vi "OAT Cascade Plot.vi"(0 "spectral map":dbl[][](array[numeric]) format="%.2f", 1 "cascade plot ref":refnum<vi>, 2 "reset? (F)":bool, 5 "spectral map info":T1={"scales"={"x scale"={"offset"=0.0, "multiplier"=0.0}, "y scale"={"offset"=0.0, "multiplier"=0.0}}, "unit labels"={"x-axis unit label"="", "y-axis unit label"="", "z-axis unit label"=""}, "plot type"=enum."Frequency-Time", "dB on"=TRUE} {"scales"."y scale"."multiplier" format="%.2f"; "scales"."y scale"."offset" format="%.2f"; "scales"."x scale"."multiplier" format="%.2f"; "scales"."x scale"."offset" format="%.2f"}, 9 "order grids to display [order]":dbl[](array[numeric]), 11 "error in (no error)":errorcluster, 12 "plot settings":T2={"plot color"=16860, "grid color"=11776947, "max Z range"=11, "number of spectra"=40} {"max Z range" items=["10^-7", "10^-6", "10^-5", "0.0001", "0.001", "0.01", "0.1", "1", "10", "100", "1000", "auto z range"]}) -> (4 "cascade plot":T3, 15 "error out":errorcluster)   [LabVIEW 2017]
doc: "LabVIEW no longer supports this VI. Use the OAT Spectral Map VI instead. Receives <B>spectral map</B> from the OAT Spectral Map VI and continuously displays the spectral lines as a function of rotational speed in a cascade plot."
uses:
  <vilib>/addons/Sound and Vibration/Order Analysis/Backward Compatibility/SubVIs/OAT Cascade Plot.ctl
  <vilib>/addons/Sound and Vibration/Order Analysis/Resample Order Tracking/SubVIs/Spectral Map Info.ctl
  <vilib>/addons/Sound and Vibration/Order Analysis/Resample Order Tracking/SoundVib_Resampling.lvlib
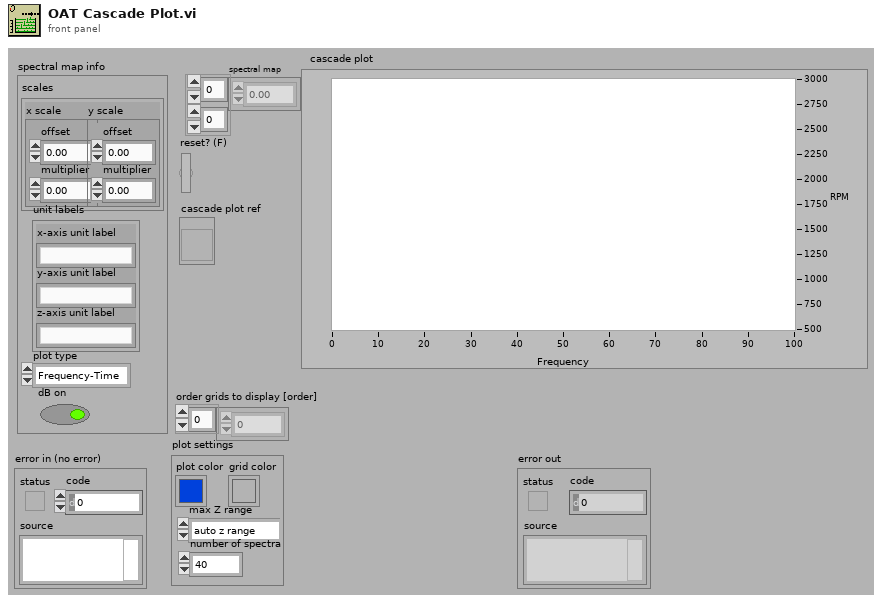
[diagram p1: front panel]
types:
  T1 = typedef "SoundVib_Resampling.lvlib/Spectral Map Info.ctl" = cluster{"scales":cluster{"x scale":cluster{"offset":dbl, "multiplier":dbl}, "y scale":cluster{"offset":dbl, "multiplier":dbl}}, "unit labels":cluster{"x-axis unit label":string, "y-axis unit label":string, "z-axis unit label":string}, "plot type":enum16{"Frequency-Time", "Time-Frequency", "Order-Time", "Time-Order", "Frequency-RPM", "RPM-Frequency", "Order-RPM", "RPM-Order"}, "dB on":bool}
  T2 = cluster{"plot color":u32, "grid color":u32, "max Z range":u16, "number of spectra":i32}
  T3 = typedef "OAT Cascade Plot.ctl" = cluster{"X0":dbl, "dX":dbl, "Y":dbl[]}[]
  T4 = cluster{"x scale":cluster{"offset":dbl, "multiplier":dbl}, "y scale":cluster{"offset":dbl, "multiplier":dbl}}
  T5 = cluster{"x-axis unit label":string, "y-axis unit label":string, "z-axis unit label":string}
  T6 = enum16{"Frequency-Time", "Time-Frequency", "Order-Time", "Time-Order", "Frequency-RPM", "RPM-Frequency", "Order-RPM", "RPM-Order"}
  T7 = cluster{"plot color":u32, "grid color":u32, dbl, "max Z range":u16, "number of spectra":i32}
  T8 = cluster{"num of displayed spectra":i32, "num of new spectra":i32}
  T9 = cluster{"plot color":u32, "grid color":u32, "X shift (rel to total X)":dbl, "max Z range":u16, "number of spectra":i32}
  T10 = cluster{"Name":string, "Color":u32, "Style":u8, "Point Style":i32, "Name Visible":bool, "Allow Drag":bool, "Lock Style":i32, "Plot":u32, "Index":i32, "Position":cluster{"X":dbl, "Y":dbl}}[]
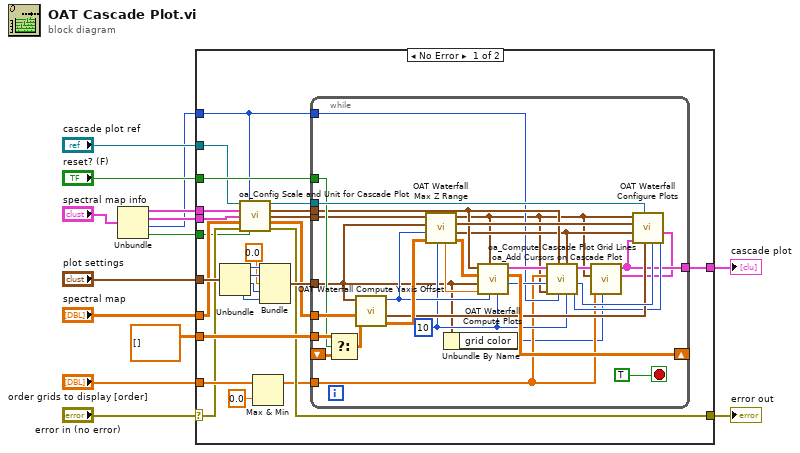
[diagram p0: block diagram]
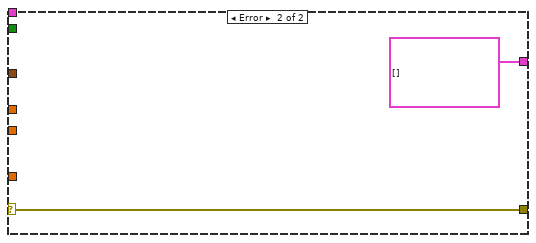
[diagram p2: hidden frame]
diagram:
  n1 = Unbundle("spectral map info") -> ("scales"=w4:T4, "unit labels"=w3:T5, "plot type"=w2:T6, "dB on"=w1:bool)
  n2 = case shown="No Error" "error in (no error)" {
    selector: "error in (no error)" -> [w19 w71]
    tunnel: w4 -> [w36 _]
    tunnel: "spectral map" -> [w23 _]
    tunnel: "reset? (F)" -> [w39 _]
    tunnel: dbl[][] [] ("spectral map") -> [w38 _]
    tunnel: "plot settings" -> [w30 _]
    tunnel: "cascade plot ref" -> [w35 _]
    tunnel: w3 -> [w34 _]
    tunnel: [w18 w71] -> w9
    tunnel: [w37 cluster{"X0":dbl, "dX":dbl, "Y":dbl[]}[] [] ("waterfall plot")] -> w8
    tunnel: w2 -> [w20 _]
    tunnel: "order grids to display [order]" -> [w31 _]
    tunnel: w1 -> [w17 _]
    frame No Error {
      n3 = Unbundle(w30) -> ("plot color"=w29:u32, "grid color"=w28:u32, "max Z range"=w24:u16, "number of spectra"=w25:i32)
      n4 = call <vilib>:"oa_Config Scale and Unit for Cascade Plot.vi"("cascade plot ref"=w35, "plot type"=w20, "scales"=w36, "unit labels"=w34, "spectral map"=w23, "error in (no error)"=w19, "dB on"=w17) -> ("cascade plot ref out"=w21:refnum<vi>, "X scale"=w32:cluster{"offset":dbl, "multiplier":dbl}, "Y scale"=w33:cluster{"offset":dbl, "multiplier":dbl}, "spectral map out"=w22:dbl[][], "error out"=w18:errorcluster)  [unwired: 4 in]
      n5 = Max & Min(x=w31, y=0.0) -> (max(x,y)=w16:dbl[])  [unwired: 1 out]
      n6 = Bundle("plot color"=w29, "grid color"=w28, 0.0, "max Z range"=w24, "number of spectra"=w25) -> (w26:T7)  [unwired: 1 in]
      n7 = while {
        shift-right: [w66] -> _
        shift-left: _ -> [w69]
        tunnel: w22 -> [w64]
        tunnel: w39 -> [w59]
        tunnel: w38 -> [w67]
        tunnel: w26 -> [w43]
        tunnel: w21 -> [w63]
        tunnel: [w45] -> w37
        tunnel: w33 -> [w49]
        tunnel: w32 -> [w56]
        tunnel: w16 -> [w44]
        tunnel: w20 -> [w52]
        stop <- TRUE stop-if-true
        w47 = 10 ("zoom factor")
        n8 = Select(t=w67, s=w59, f=w69) -> (s? t:f=w65:dbl[][])
        n9 = call <vilib>:"OAT Waterfall Compute Yaxis Offset.vi"("spectral map history"=w65, "spectral map new"=w64, "plot settings"=w43) -> ("spectral map for display"=w62:dbl[][], "spectra info"=w50:T8, "Y axis offset"=w57:i32)  [unwired: 6 in]
        n10 = call <vilib>:"OAT Waterfall Max Z Range.vi"("zoom factor"=w47, "spectral map in"=w62, "Y axis offset"=w57, "plot settings"=w43, "scale in"=w49) -> ("spectral map out"=w61:dbl[][], "Y range"=w55:cluster{"min":dbl, "max":dbl}, "plot settings"=w60:T9, "scale out"=w41:cluster{"offset":dbl, "multiplier":dbl}, "max Z range"=w54:dbl)  [unwired: 2 in]
        n11 = Unbundle By Name(w43) -> ("grid color"=w42:u32)
        n12 = call <vilib>:"OAT Waterfall Compute Plots.vi"("zoom factor"=w47, "Y axis offset"=w57, "Y scale"=w41, "max Z range"=w54, "plot settings"=w43, "spectral map in"=w61, "X scale"=w56) -> ("# of bins"=w53:i32, "spectral map out"=w66:dbl[][], "waterfall plot"=w58:cluster{"X0":dbl, "dX":dbl, "Y":dbl[]}[])  [unwired: 1 in, 1 out]
        n13 = call <vilib>:"oa_Compute Cascade Plot Grid Lines.vi"("zoom factor"=w47, "Y range"=w55, "plot type"=w52, "X scale"=w56, "Y scale"=w41, "# of bins"=w53, "grid lines to plot [Hz/Order]"=w44, "waterfall plot"=w58) -> ("# of axis lines"=w48:i32, "# of grid lines"=w51:i32, "waterfall plot out"=w46:cluster{"X0":dbl, "dX":dbl, "Y":dbl[]}[])  [unwired: 1 in]
        n14 = call <vilib>:"oa_Add Cursors on Cascade Plot.vi"("grid color"=w42, "order grids to display [order]"=w44, "Y scale"=w41, "waterfall plot"=w46) -> ("cursor list"=w40:T10, "waterfall plot out"=w45:cluster{"X0":dbl, "dX":dbl, "Y":dbl[]}[])  [unwired: 6 in]
        n15 = call <vilib>:"OAT Waterfall Configure Plots.vi"("# of axis lines"=w48, "cursor list"=w40, "# of grid lines"=w51, "spectra info"=w50, "reference"=w63, "waterfall plot"=w45, "Y range"=w55, "plot settings"=w60, "Y scale"=w41) -> ()  [unwired: 2 in, 1 out]
      }
    }
    frame Error {
    }
  }
  "cascade plot" <- w8
  "error out" <- w9
